vi "INTELLIFAUCET TEMPFLOW Contact Tester.vi"(8 "error in (no error)":errorcluster, 9 "MicroAmp":i32, 10 "TEMP,FLOW":T1=enum."FLOW", 11 "VISA Refnum in":refnum<visa-resource-name>) -> (0 "error out":errorcluster, 3 "VISA Refnum out":refnum<visa-resource-name>)   [LabVIEW 2016]
uses:
  Type Definitions/INTELLIFAUCT Temp Flow.ctl
  MW100/Type Definitions/HEWH MW100 Channel Numbers.ctl
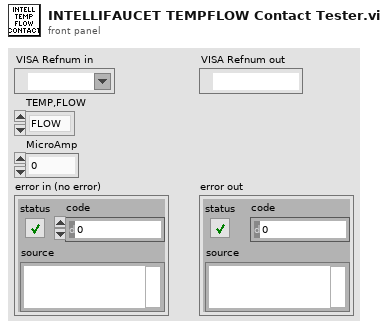
[diagram p1: front panel]
types:
  T1 = typedef "INTELLIFAUCT Temp Flow.ctl" = enum8{"TEMP", "FLOW"}
  T2 = typedef "HEWH MW100 Channel Numbers.ctl" = string
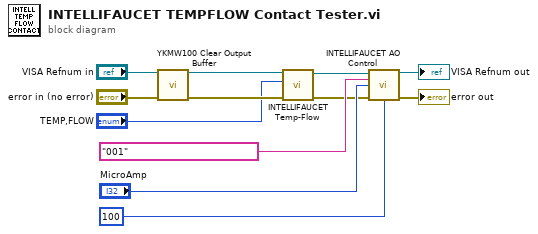
[diagram p0: block diagram]
diagram:
  n1 = call "YKMW100 Clear Output Buffer.vi"("VISA session"="VISA Refnum in", "error in (no error)"="error in (no error)") -> ("dup VISA session"=w6:refnum<visa-resource-name>, "error out"=w5:errorcluster)  [unwired: 12 in]
  n2 = call "INTELLIFAUCET Temp-Flow.vi"("Error In"=w5, "TEMP,FLOW"="TEMP,FLOW", "VISA session"=w6) -> ("Error Out"=w7:errorcluster, "dup VISA session"=w9:refnum<visa-resource-name>)  [unwired: 7 in]
  n3 = call "INTELLIFAUCET AO Control.vi"("VISA session"=w9, "HEWH MW100 Channel Numbers"=T2 "001", "Output Value (0)"="MicroAmp", "Error In"=w7, "milliseconds to wait"=u32 100) -> ("dup VISA session"=→"VISA Refnum out":refnum<visa-resource-name>, "error out"=→"error out":errorcluster)  [unwired: 9 in]
